vi "WPI_UtilitiesRebuildVariableName.vi"(10 "Test Tree":string, 11 "TreeControl in":refnum<vi>) -> (3 "Variable Name":string)   [LabVIEW 2019]
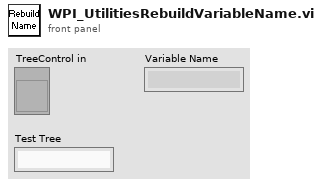
[diagram p1: front panel]
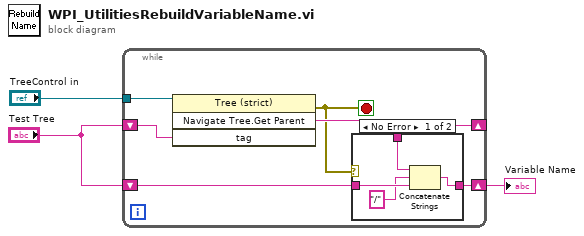
[diagram p0: block diagram]
diagram:
  n1 = while {
    tunnel: "TreeControl in" -> [w9]
    shift-right: [w5] -> _
    shift-left: "Test Tree" -> [w6]
    shift-right: [w7] -> w2
    shift-left: "Test Tree" -> [w8]
    stop <- w4 stop-if-true
    n2 = invoke on="Invoke Node" class="Tree (strict)" method="Navigate Tree.Get Parent"(reference=w9, "tag"=w6) -> (error out=w4:errorcluster, "Navigate Tree:Get Parent"=w5:string)  [unwired: 2 in, 2 out]
    n3 = case shown="No Error" w4 {
      tunnel: w8 -> [w13 w14]
      tunnel: [w12 w14] -> w7
      tunnel: w5 -> [w10 _]
      frame No Error {
        n4 = Concatenate Strings(w10, "/", w13) -> (w12:string)
      }
      frame Error {
      }
    }
  }
  "Variable Name" <- w2
